vi "Create FIFO.vi"(8 "error in (no error)":errorcluster, 10 "DataRef":T3 {"Block Data Refs"."Data Reference" format="%.0x"}, 11 "FIFO Name":string="Write SV") -> (0 "error out":errorcluster, 3 "FIFO Ref":refnum<k33>)   [LabVIEW 2017, in "Shared Variables CD 2.0 Engine.lvlib"]
uses:
  <vilib>/NI Veristand/Custom Device API/Block Data Reference.ctl
  <vilib>/NI Veristand/Custom Device API/Data Reference.ctl
  Shared Variables CD 2.0 Engine.lvlib
  <vilib>/NI Veristand/Custom Device API/Custom Device API.lvlib
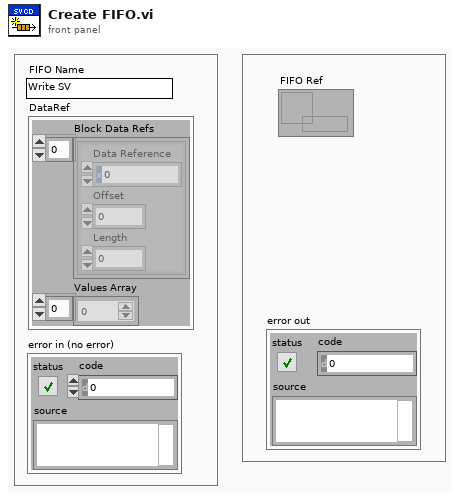
[diagram p1: front panel]
types:
  T1 = typedef "Custom Device API.lvlib/Block Data Reference.ctl" = cluster{"Data Reference":T2, "Offset":u64, "Length":u64}
  T2 = typedef "Custom Device API.lvlib/Data Reference.ctl" = i32
  T3 = cluster{"Block Data Refs":T1[], "Values Array":dbl[]}
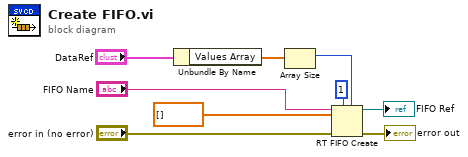
[diagram p0: block diagram]
diagram:
  n1 = Unbundle By Name("DataRef") -> ("Values Array"=w1:dbl[])
  n2 = Array Size(array=w1) -> (size(s)=w3:i32)
  n3 = RT FIFO Create(0:"FIFO Name", 1:dbl[] [] ("Output Values"), 3:"error in (no error)", 4:u32 1 ("size (10)"), 6:w3) -> (8:→"FIFO Ref":refnum<k33>, 11:→"error out":errorcluster)  [unwired: 3 in, 1 out]
